vi "fpga_ErrorCode.vi"(4 "resampling FIFO time in":bool=TRUE, 6 "Ref filter FIFO time in":bool=TRUE, 9 "samples per cycle":u16=192, 10 "reference channel index":u8, 11 "number of channels":u8) -> (0 "error":i32, 1 "samples per cycle out":u16, 2 "ref channel index out":u8, 3 "number of CH out":u8)   [LabVIEW 2011, in "NI_EP_Resample_FPGA.lvlib"]
uses:
  <vilib>/addons/Electrical Power/PQ/Resampling/NI_EP_Resample_FPGA.lvlib
panel:
  out "Ref filter FIFO time out":bool=TRUE
  out "resampling FIFO time out":bool=TRUE
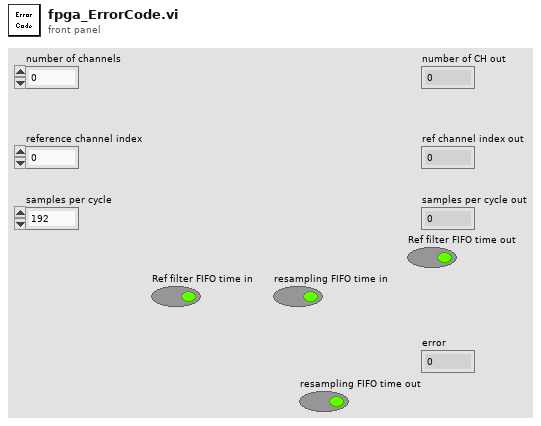
[diagram p1: front panel]
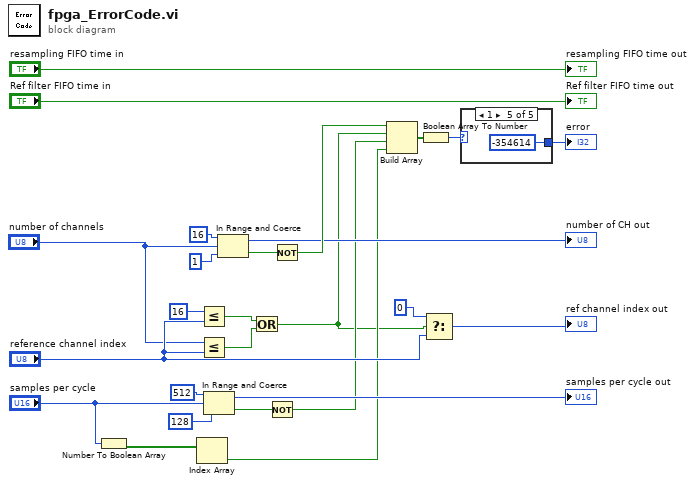
[diagram p0: block diagram]
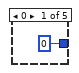
[diagram p2: hidden frame]
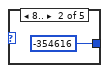
[diagram p3: hidden frame]
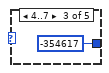
[diagram p4: hidden frame]
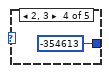
[diagram p5: hidden frame]
diagram:
  n1 = Number To Boolean Array(number="samples per cycle") -> (Boolean array=w13:bool[])
  n2 = Index Array(array=w13) -> (element=w5:bool)  [unwired: 1 in]
  n3 = Less Or Equal?(x=u8 16, y="reference channel index") -> (x <= y?=w19:bool)
  n4 = Less Or Equal?(x="number of channels", y="reference channel index") -> (x <= y?=w18:bool)
  n5 = In Range and Coerce(upper limit=u16 512, x="samples per cycle", lower limit=u16 128) -> (coerced(x)=→"samples per cycle out":u16, In Range?=w12:bool)
  n6 = In Range and Coerce(upper limit=u8 16 ("x"), x="number of channels", lower limit=u8 1 ("x")) -> (coerced(x)=→"number of CH out":u8, In Range?=w8:bool)
  n7 = Or(x=w19, y=w18) -> (x .or. y?=w1:bool)
  n8 = Not(x=w12) -> (.not. x?=w4:bool)
  n9 = Not(x=w8) -> (.not. x?=w7:bool)
  n10 = Build Array(w7, w1, w4, w5) -> (w24:bool[])
  n11 = Boolean Array To Number(Boolean array=w24) -> (number=w3:u8)
  n12 = Select(t=u8 0 ("x"), s=w1, f="reference channel index") -> (s? t:f=→"ref channel index out":u8)
  n13 = case shown="1" w3 {
    tunnel: [0 ("error") -354616 ("error") -354617 ("error") -354613 ("error") -354614 ("error")] -> w2
    frame 0 {
    }
    frame 8.. {
    }
    frame 4..7 {
    }
    frame 2, 3 {
    }
    frame 1 {
    }
  }
  "error" <- w2
  "resampling FIFO time out" <- "resampling FIFO time in"
  "Ref filter FIFO time out" <- "Ref filter FIFO time in"
